vi "Pot Line of Lines.vi"(6 "Potting Parameters":T1={"Curing Param A"=0.0, "Curing Param B"=0.0, "Speed Nominal"=-1.0, "Time Nominal"=0.0, "Turn-on Time"=0.0, "Turn-off Time"=0.0, "Safe Height Offset"=0.0, "Tip Height"=0.0, "Width of Line"=0.0, "Number of lines"=1.0, "Distance between lines"=0.0}, 7 "Potting Surface Type":T2, 8 "error in (no error)":errorcluster, 9 "End Position":refnum<class "Vec3d Class.lvclass">, 10 "Start Position":refnum<class "Vec3d Class.lvclass">, 11 "SyringeTool Class in":refnum<class "SyringeTool Class.lvclass">) -> (0 "error out":errorcluster, 3 "SyringeTool Class out":refnum<class "SyringeTool Class.lvclass">)   [LabVIEW 2017, in "SyringeTool Class.lvclass"]
uses:
  SyringeTool Class.lvclass
  Config Manager Class/Type Definitions/Potting Surface Type.ctl
  Vec3d Class/Vec3d Class.lvclass
  Config Manager Class/Type Definitions/Potting Parameters.ctl
  Utils/Type Definitions/3d Line.ctl
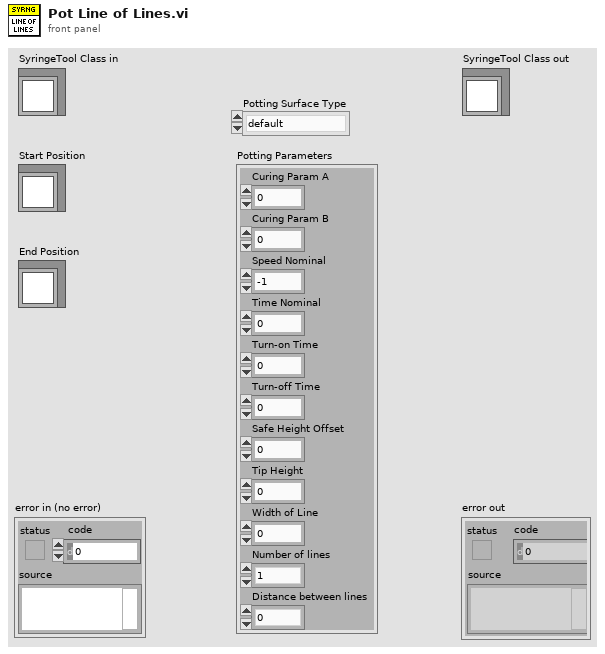
[diagram p1: front panel]
types:
  T1 = typedef "Potting Parameters.ctl" = cluster{"Curing Param A":dbl, "Curing Param B":dbl, "Speed Nominal":dbl, "Time Nominal":dbl, "Turn-on Time":dbl, "Turn-off Time":dbl, "Safe Height Offset":dbl, "Tip Height":dbl, "Width of Line":dbl, "Number of lines":dbl, "Distance between lines":dbl}
  T2 = typedef "Potting Surface Type.ctl" = enum16{"default", "hdi_edge_pads", "bbm_edge_pads", "address_pads"}
  T3 = typedef "3d Line.ctl" = cluster{"Start":refnum<class "Vec3d Class.lvclass">, "End":refnum<class "Vec3d Class.lvclass">, "Enable":bool}
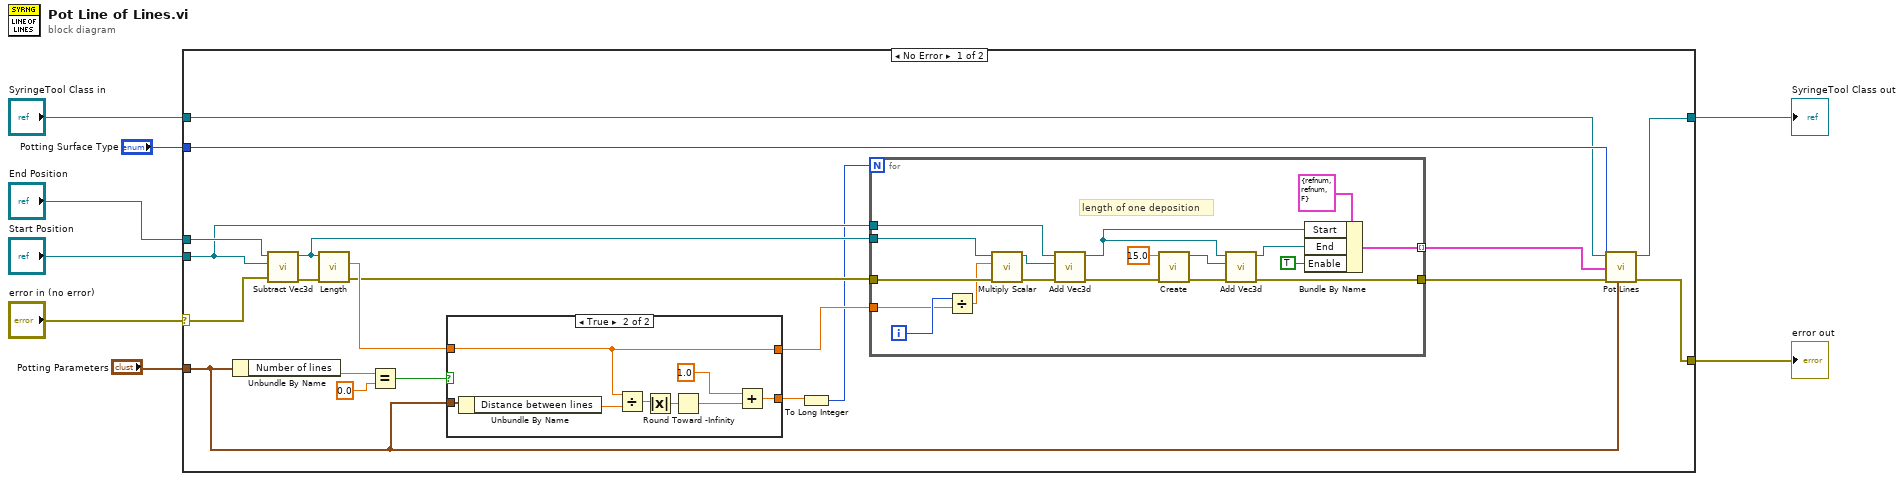
[diagram p0: block diagram]
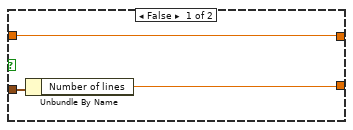
[diagram p2: hidden frame]
diagram:
  n1 = case shown="No Error" "error in (no error)" {
    selector: "error in (no error)" -> [w22 w59]
    tunnel: [w19 w58] -> w6
    tunnel: "SyringeTool Class in" -> [w20 w58]
    tunnel: "Start Position" -> [w17 _]
    tunnel: "End Position" -> [w18 _]
    tunnel: "Potting Surface Type" -> [w23 _]
    tunnel: [w21 w59] -> w4
    tunnel: "Potting Parameters" -> [w9 _]
    frame No Error {
      n2 = Unbundle By Name(w9) -> ("Number of lines"=w16:dbl)
      n3 = call "Subtract Vec3d.vi"("error in (no error)"=w22, "Vec3d in 2"=w17, "Vec3d in 1"=w18) -> ("error out"=w28:errorcluster, "Vec3d Class out"=w27:refnum<class "Vec3d Class.lvclass">)  [unwired: 7 in]
      n4 = call-dynamic "Length.vi"("error in"=w28, "Vec3d in"=w27) -> ("error out"=w25:errorcluster, "Length"=w26:dbl)  [unwired: 7 in, 1 out]
      n5 = Equal?(x=w16, y=0.0) -> (x = y?=w14:bool)
      n6 = case shown="True" w14 {
        tunnel: w26 -> [w47 w50]
        tunnel: w9 -> [w49 w55]
        tunnel: [w48 w51] -> w11
        tunnel: [w47 w50] -> w13
        frame False {
          n7 = Unbundle By Name(w49) -> ("Number of lines"=w48:dbl)
        }
        frame True {
          n8 = Unbundle By Name(w55) -> ("Distance between lines"=w54:dbl)
          n9 = Divide(x=w50, y=w54) -> (x/y=w56:dbl)
          n10 = Absolute Value(x=w56) -> (abs(x)=w57:dbl)
          n11 = Round Toward -Infinity(1:w57) -> (0:w52:dbl)
          n12 = Add(x=1.0, y=w52) -> (x+y=w51:dbl)
        }
      }
      n13 = To Long Integer(number=w11) -> (32bit integer=w12:i32)
      n14 = for {
        N: w12 -> [_]
        tunnel: [w46] -> w10 mode=indexing
        tunnel: w27 -> [w45]
        tunnel: w25 -> [w44]
        tunnel: [w29] -> w24
        tunnel: w17 -> [w42]
        tunnel: w13 -> [w38]
        i -> [w39]
        # "length of one deposition"
        n15 = Divide(x=w39, y=w38) -> (x/y=w40:dbl)
        n16 = call-dynamic "Multiply Scalar.vi"("error in"=w44, "Scale"=w40, "Vec3d in"=w45) -> ("error out"=w43:errorcluster, "Vec3d out"=w41:refnum<class "Vec3d Class.lvclass">)  [unwired: 7 in]
        n17 = call-dynamic "Add Vec3d.vi"("error in (no error)"=w43, 10:"Vec3d Class in"=w41, 11:"Vec3d Class in"=w42) -> ("error out"=w33:errorcluster, "Vec3d Class out"=w31:refnum<class "Vec3d Class.lvclass">)  [unwired: 7 in]
        n18 = call "Create.vi"("error in"=w33, "X"=15.0) -> ("error out"=w30:errorcluster, "Vec3d Class out"=w34:refnum<class "Vec3d Class.lvclass">)  [unwired: 8 in]
        n19 = call-dynamic "Add Vec3d.vi"("error in (no error)"=w30, 10:"Vec3d Class in"=w34, 11:"Vec3d Class in"=w31) -> ("error out"=w29:errorcluster, "Vec3d Class out"=w35:refnum<class "Vec3d Class.lvclass">)  [unwired: 7 in]
        n20 = Bundle By Name(cluster=T3 {"Start"=refnum, "End"=refnum, "Enable"=FALSE} ("Cluster"), "Start"=w31, "End"=w35, "Enable"=TRUE) -> (w46:T3)
      }
      n21 = call-dynamic "Pot Lines.vi"("Potting Parameters"=w9, "Potting Surface Type"=w23, "error in"=w24, "Potting Lines"=w10, "SyringeTool in"=w20) -> ("error out"=w21:errorcluster, "SyringeTool out"=w19:refnum<class "SyringeTool Class.lvclass">)  [unwired: 5 in]
    }
    frame Error {
    }
  }
  "error out" <- w4
  "SyringeTool Class out" <- w6
